vi "S2C_FPGA_WriteIsoConn.vi"(11 "Reset":bool) -> ()   [LabVIEW 2015]
uses:
  S2C_FPGA_Global.vi
  <vilib>/rvi/eio/common/nirviEmuTemplateMethod_errors.vi
  <vilib>/eio/EIONode/EIONode.xnode
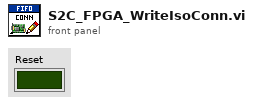
[diagram p1: front panel]
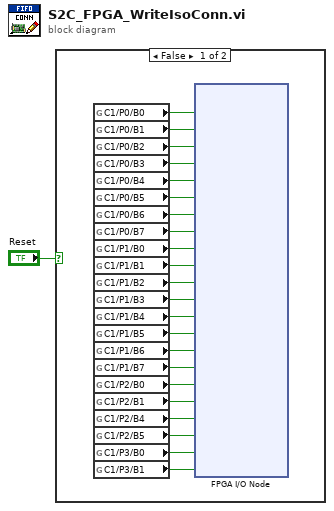
[diagram p0: block diagram]
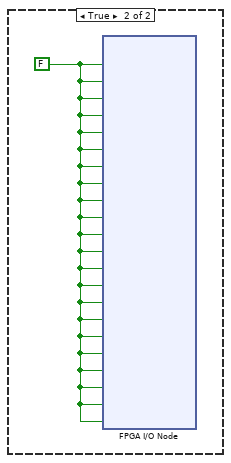
[diagram p2: hidden frame]
diagram:
  n1 = case shown="False" "Reset" {
    frame False {
      n2 = global read "S2C_FPGA_Global.vi" "C1/P0/B0"() -> (w23:bool)
      n3 = global read "S2C_FPGA_Global.vi" "C1/P0/B1"() -> (w22:bool)
      n4 = global read "S2C_FPGA_Global.vi" "C1/P0/B2"() -> (w21:bool)
      n5 = global read "S2C_FPGA_Global.vi" "C1/P0/B3"() -> (w20:bool)
      n6 = global read "S2C_FPGA_Global.vi" "C1/P0/B4"() -> (w19:bool)
      n7 = global read "S2C_FPGA_Global.vi" "C1/P0/B5"() -> (w18:bool)
      n8 = global read "S2C_FPGA_Global.vi" "C1/P0/B6"() -> (w17:bool)
      n9 = global read "S2C_FPGA_Global.vi" "C1/P0/B7"() -> (w16:bool)
      n10 = global read "S2C_FPGA_Global.vi" "C1/P1/B0"() -> (w15:bool)
      n11 = global read "S2C_FPGA_Global.vi" "C1/P1/B1"() -> (w14:bool)
      n12 = global read "S2C_FPGA_Global.vi" "C1/P1/B2"() -> (w13:bool)
      n13 = global read "S2C_FPGA_Global.vi" "C1/P1/B3"() -> (w12:bool)
      n14 = global read "S2C_FPGA_Global.vi" "C1/P1/B4"() -> (w11:bool)
      n15 = global read "S2C_FPGA_Global.vi" "C1/P1/B5"() -> (w10:bool)
      n16 = global read "S2C_FPGA_Global.vi" "C1/P1/B6"() -> (w9:bool)
      n17 = global read "S2C_FPGA_Global.vi" "C1/P1/B7"() -> (w8:bool)
      n18 = global read "S2C_FPGA_Global.vi" "C1/P2/B0"() -> (w7:bool)
      n19 = global read "S2C_FPGA_Global.vi" "C1/P2/B1"() -> (w6:bool)
      n20 = global read "S2C_FPGA_Global.vi" "C1/P2/B4"() -> (w5:bool)
      n21 = global read "S2C_FPGA_Global.vi" "C1/P2/B5"() -> (w4:bool)
      n22 = global read "S2C_FPGA_Global.vi" "C1/P3/B0"() -> (w3:bool)
      n23 = global read "S2C_FPGA_Global.vi" "C1/P3/B1"() -> (w2:bool)
      n24 = xnode "FPGA I/O Node"("C1/P0/B0"=w23, "C1/P0/B1"=w22, "C1/P0/B2"=w21, "C1/P0/B3"=w20, "C1/P0/B4"=w19, "C1/P0/B5"=w18, "C1/P0/B6"=w17, "C1/P0/B7"=w16, "C1/P1/B0"=w15, "C1/P1/B1"=w14, "C1/P1/B2"=w13, "C1/P1/B3"=w12, "C1/P1/B4"=w11, "C1/P1/B5"=w10, "C1/P1/B6"=w9, "C1/P1/B7"=w8, "C1/P2/B0"=w7, "C1/P2/B1"=w6, "C1/P2/B4"=w5, "C1/P2/B5"=w4, "C1/P3/B0"=w3, "C1/P3/B1"=w2) -> ()  [unwired: 22 in, 22 out]
    }
    frame True {
      w24 = FALSE ("C2/P0/B0")
      n25 = xnode "FPGA I/O Node"("C1/P0/B0"=w24, "C1/P0/B1"=w24, "C1/P0/B2"=w24, "C1/P0/B3"=w24, "C1/P0/B4"=w24, "C1/P0/B5"=w24, "C1/P0/B6"=w24, "C1/P0/B7"=w24, "C1/P1/B0"=w24, "C1/P1/B1"=w24, "C1/P1/B2"=w24, "C1/P1/B3"=w24, "C1/P1/B4"=w24, "C1/P1/B5"=w24, "C1/P1/B6"=w24, "C1/P1/B7"=w24, "C1/P2/B0"=w24, "C1/P2/B1"=w24, "C1/P2/B4"=w24, "C1/P2/B5"=w24, "C1/P3/B0"=w24, "C1/P3/B1"=w24) -> ()  [unwired: 22 in, 22 out]
    }
  }
